vi "Test Comment AE.vi"() -> ()   [LabVIEW 2016, in "User Interface.lvlib"]
uses:
  User Interface.lvlib
  Test Data.ctl
  Create Path Command.ctl
  <vilib>/Utility/xml.llb/Write to XML File(string).vi
  <vilib>/Utility/xml.llb/Read From XML File(array).vi
  Test Comment Command.ctl
panel:
  out "Test Details":T1(array[cluster])
  out "XML Elements":string[](array[string])
  in  "Comm":T2
  out "error out":errorcluster
  in  "error in (no error)":errorcluster
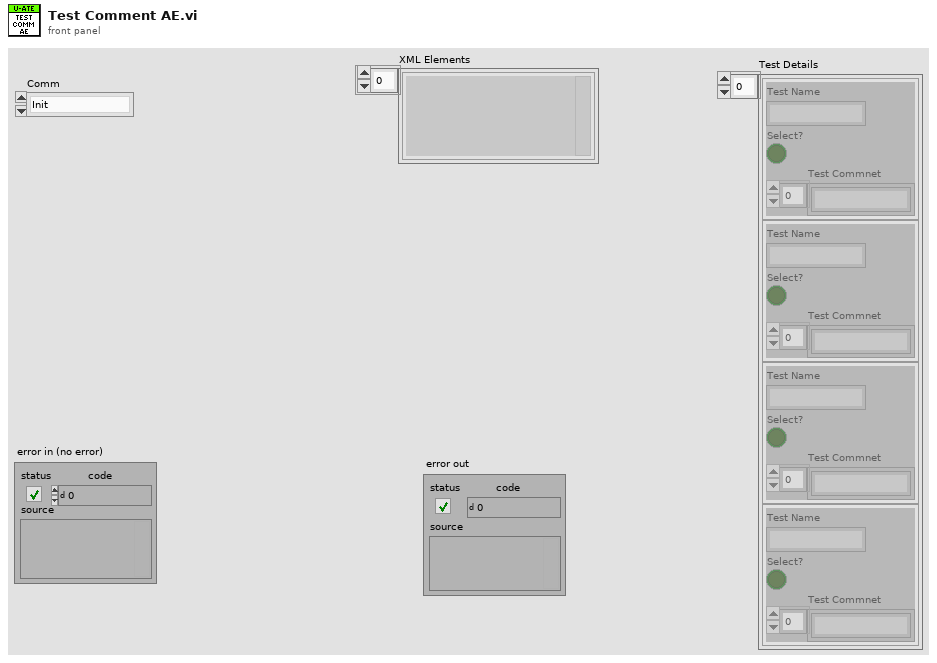
[diagram p1: front panel]
types:
  T1 = cluster{"Test Name":string, "Select?":bool, "Test Commnet":string[]}[]
  T2 = typedef "User Interface.lvlib/Test Comment Command.ctl" = enum16{"Init", "Read", "Write", "Close"}
  T3 = typedef "User Interface.lvlib/Test Data.ctl" = cluster{"Test Details":cluster{"Test Name":string, "Select?":bool, "Test Commnet":string[]}[], "Test Description Path":path}
  T4 = typedef "User Interface.lvlib/Create Path Command.ctl" = enum16{"Authentication", "Hardware", "Configuration", "Calibration", "Instrument", "Test Description", "Serial Data", "ARINC Data", "CAN Data", "Data", "Report", "Action log", "Error Log"}
  T5 = cluster{"Test Name":string, "Select?":bool, "Test Commnet":string[]}
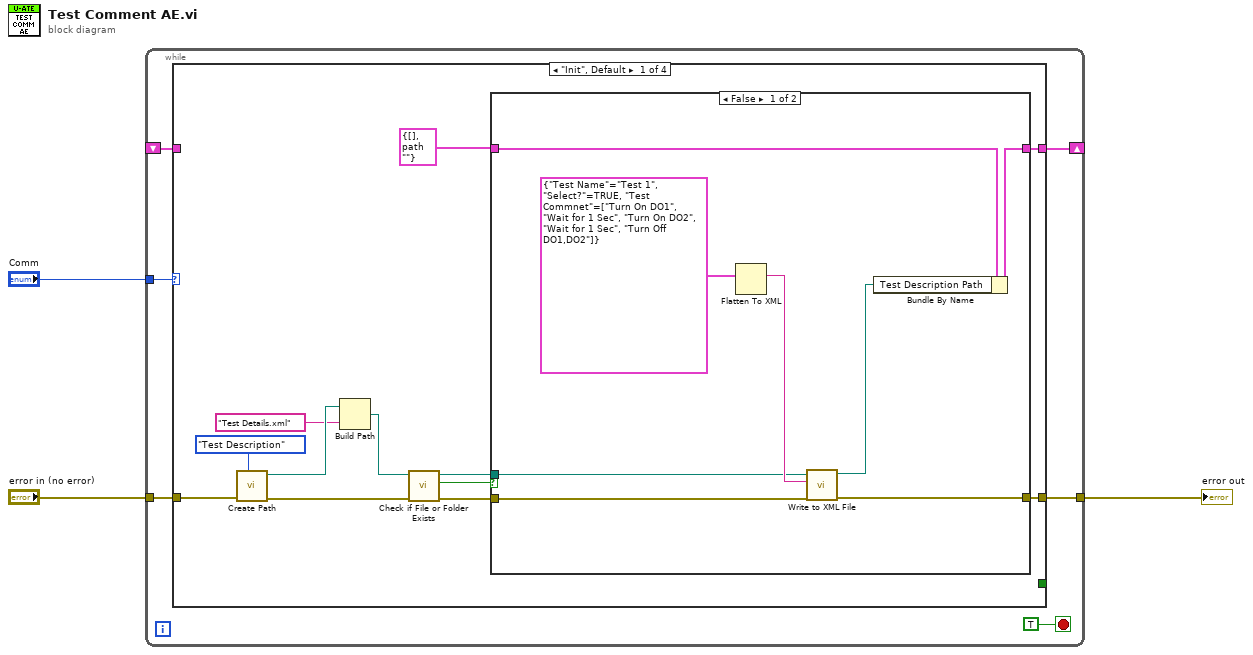
[diagram p0: block diagram]
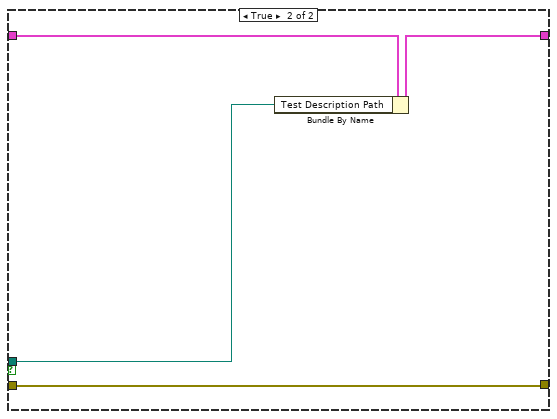
[diagram p2: hidden frame]
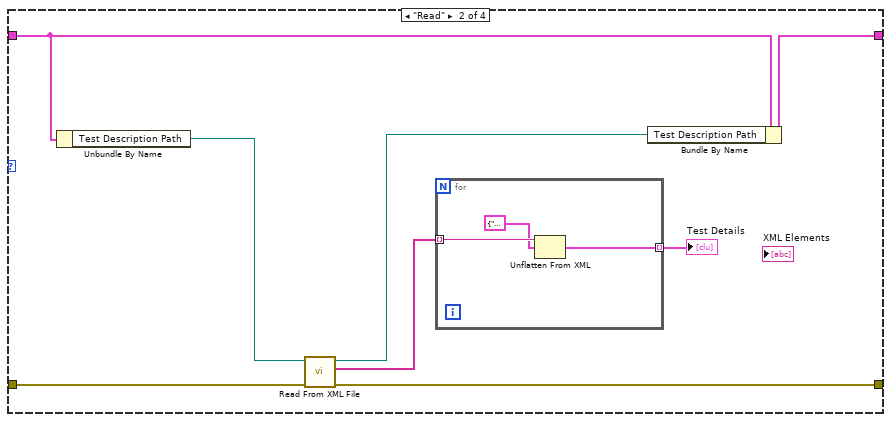
[diagram p3: hidden frame]
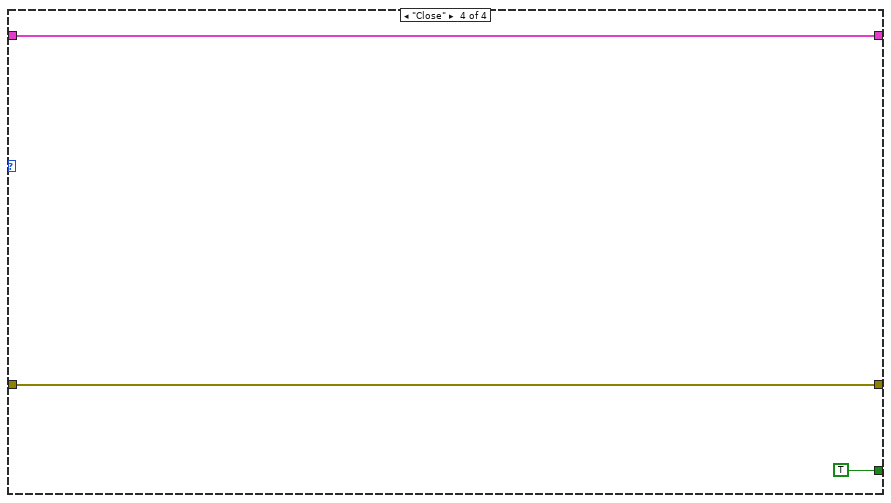
[diagram p5: hidden frame]
diagram:
  n1 = while {
    tunnel: "Comm" -> [w9]
    tunnel: "error in (no error)" -> [w8]
    tunnel: [w7] -> w1
    shift-right: [w5] -> _
    shift-left: _ -> [w6]
    stop <- TRUE stop-if-true
    n2 = case shown="\"Init\", Default" w9 {
      tunnel: [_ _ _ TRUE] -> _
      tunnel: w8 -> [w21 w41 _ w47]
      tunnel: [w11 w40 _ w47] -> w7
      tunnel: w6 -> [_ w39 w45 w46]
      tunnel: [w13 w37 w45 w46] -> w5
      frame "Init", Default {
        n3 = call "Create Path.vi"("Path Command"=Create_Path_Command."Test Description", "error in (no error)"=w21) -> ("error out"=w16:errorcluster, "created path"=w19:path)  [unwired: 8 in]
        n4 = Build Path(base path=w19, name or relative path="Test Details.xml") -> (appended path=w17:path)
        n5 = call <vilib>:"Check if File or Folder Exists.vi"("error in (no error)"=w16, "path"=w17) -> ("error out"=w15:errorcluster, "file or folder exists?"=w14:bool, "dup path"=w12:path)  [unwired: 7 in]
        n6 = case shown="False" w14 {
          tunnel: w15 -> [w28 w30]
          tunnel: T3 {"Test Details"=[], "Test Description Path"=path ""} -> [w29 w33]
          tunnel: [w24 w32] -> w13
          tunnel: w12 -> [w26 w31]
          tunnel: [w25 w30] -> w11
          frame False {
            n7 = Flatten To XML(anything=T5 {"Test Name"="Test 1", "Select?"=TRUE, "Test Commnet"=["Turn On DO1", "Wait for 1 Sec", "Turn On DO2", "Wait for 1 Sec", "Turn Off DO1,DO2"]} ("Test Info")) -> (xml string=w27:string)
            n8 = call-poly <vilib>:"Write to XML File.vi"("error in (no error)"=w28, "XML Input"=w27, "XML File Path"=w26) -> ("error out"=w25:errorcluster, "XML File Path(duplicate)"=w23:path)  [unwired: 6 in, 1 out]
            n9 = Bundle By Name(cluster=w29, "Test Description Path"=w23) -> (w24:T3)
          }
          frame True {
            n10 = Bundle By Name(cluster=w33, "Test Description Path"=w31) -> (w32:T3)
          }
        }
      }
      frame "Read" {
        n11 = Unbundle By Name(w39) -> ("Test Description Path"=w38:path)
        n12 = call-poly <vilib>:"Read From XML File.vi"("error in (no error)"=w41, "XML File Path"=w38) -> ("error out"=w40:errorcluster, "XML Elements"=w35:string[], "XML File Path(duplicate)"=w36:path)  [unwired: 7 in]
        n13 = for {
          tunnel: w35 -> [w43] mode=indexing
          tunnel: [w44] -> w34 mode=indexing
          n14 = Unflatten From XML(xml string=w43, type=T5 {"Test Name"="", "Select?"=FALSE, "Test Commnet"=[]} ("Test Info")) -> (value=w44:T5)  [unwired: 1 in, 1 out]
        }
        "Test Details" <- w34
        n15 = Bundle By Name(cluster=w39, "Test Description Path"=w36) -> (w37:T3)
      }
      frame "Write" {
      }
      frame "Close" {
      }
    }
  }
  "error out" <- w1
